vi "Command Information.vi"() -> (0 "Variant":variant)   [LabVIEW 2018]
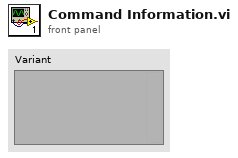
[diagram p1: front panel]
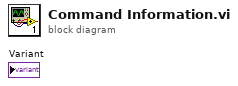
[diagram p0: block diagram]
diagram:
